vi "InterruptVoltage.vi"() -> ()   [LabVIEW 2015]
uses:
  <vilib>/myRIO/Express VI/IRQ/IRQ Express VI.xnode
  <vilib>/myRIO/Instrument Drivers/IRQ/IO IRQ/IO IRQ.lvlib
  Voltage_global.vi
  <vilib>/myRIO/Common/Instrument Driver Framework/myRIO v1.0/IRQ/typedefs/DI IRQ Type.ctl
  <vilib>/myRIO/Common/Instrument Driver Framework/myRIO v1.0/IRQ/typedefs/Callback VI Ref.ctl
  <vilib>/myRIO/Instrument Drivers/IRQ/IO IRQ/vis/myRIO Register DI IRQ.xnode
  <vilib>/myRIO/Common/Instrument Driver Framework/myRIO v1.0/IRQ/vis/myRIO v1.1 Register DI IRQ.vi
  <vilib>/userdefined/High Color/nirio_resource_hc.ctl
panel:
  in  "stop":bool
  out "Measured Voltage":dbl format="%#.2g"
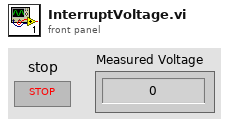
[diagram p1: front panel]
types:
  T1 = typedef "DI IRQ Type.ctl" = enum16{"Digital falling edge", "Digital rising edge", "Digital edge"}
  T2 = typedef "nirio_resource_hc.ctl" = tag
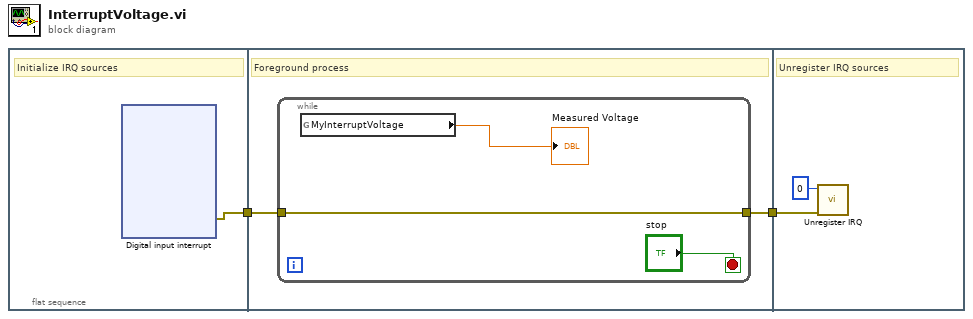
[diagram p0: block diagram]
diagram:
  n1 = flat-sequence {
    tunnel: [w3] -> w1
    tunnel: [w22] -> w2
    tunnel: w1 -> [w21]
    tunnel: w2 -> [w26]
    frame #0 {
      # "Initialize IRQ sources"
      n2 = xnode "Digital input interrupt"() -> ("error out"=w3:errorcluster)  [unwired: 1 in]
    }
    frame #1 {
      # "Foreground process"
      n3 = while {
        tunnel: w21 -> [w24]
        tunnel: [w24] -> w22
        stop <- "stop" stop-if-true
        n4 = global read "Voltage_global.vi" "MyInterruptVoltage"() -> (→"Measured Voltage":dbl)
      }
    }
    frame #2 {
      # "Unregister IRQ sources"
      n5 = call <vilib>:"Unregister IRQ.vi"("error in (no error)"=w26, "IRQ Number"=u8 0) -> ()  [unwired: 9 in, 1 out]
    }
  }
